vi "Cxns-Write Configuration (keyed on endpoints).vi"(0 "Connection File Path":path, 2 "Section":string, 5 "Outputs":string[](array[string]), 9 "Endpoints":string[](array[string]), 11 "error in (no error)":errorcluster) -> (4 "Path Out":path, 15 "error out":errorcluster)   [LabVIEW 2020]
uses:
  <vilib>/Utility/config.llb/Write Key (String).vi
  <vilib>/Utility/config.llb/NI_LVConfig.lvlib
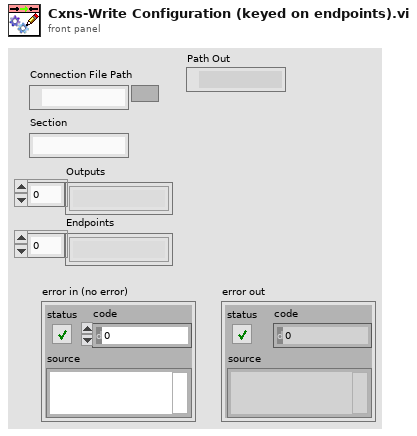
[diagram p1: front panel]
types:
  T1 = typedef "NI_LVConfig.lvlib/Config Data RefNum.ctl" = refnum<k1>
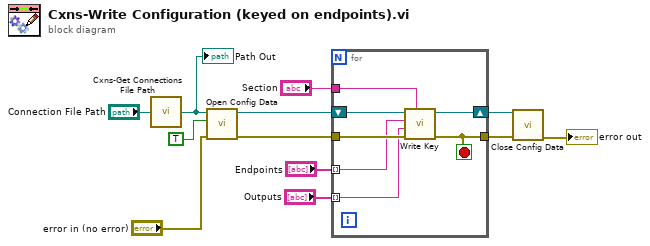
[diagram p0: block diagram]
diagram:
  n1 = call "Cxns-Get Connections File Path.vi"("Connection File Path"="Connection File Path") -> ("Path Out"=w5:path)
  "Path Out" <- w5
  n2 = call <vilib>:"Open Config Data.vi"("error in (no error)"="error in (no error)", "create file if necessary (T)"=TRUE, "configuration file path"=w5) -> ("error out"=w9:errorcluster, "refnum"=w11:T1)  [unwired: 6 in, 1 out]
  n3 = for {
    tunnel: "Endpoints" -> [w14] mode=indexing
    tunnel: "Section" -> [w18]
    tunnel: w9 -> [w17]
    tunnel: [w16] -> w8
    shift-right: [w15] -> w7
    shift-left: w11 -> [w19]
    tunnel: "Outputs" -> [w13] mode=indexing
    stop <- w16 stop-if-true
    n4 = call-poly <vilib>:"Write Key.vi"("section"=w18, "error in (no error)"=w17, "value"=w13, "key"=w14, "refnum"=w19) -> ("error out"=w16:errorcluster, "refnum out"=w15:T1)  [unwired: 4 in, 1 out]
  }
  n5 = call <vilib>:"Close Config Data.vi"("error in (no error)"=w8, "refnum"=w7) -> ("error out"=→"error out":errorcluster)  [unwired: 8 in, 1 out]
